vi "BMcalculate_v2_0.vi"() -> ()   [LabVIEW 2014]
uses:
  <vilib>/Analysis/coordinate.llb/2D Cartesian Coordinate Rotation (Array).vi
  <vilib>/Analysis/baseanly.llb/Mean (DBL).vi
  <vilib>/Utility/file.llb/Read From Spreadsheet File (string).vi
  <vilib>/Utility/file.llb/Write To Spreadsheet File (DBL).vi
  <vilib>/Analysis/NI_AALBase.lvlib
  <vilib>/Analysis/NI_AALPro.lvlib
panel:
  in  "(T=X , F=Y)":bool=TRUE
  in  "Filter window size":i32=100
  out "Array":dbl[](array[numeric])
  out "XYplot":path
  out "TimeTrace":path
  in  "Save Time-trace":bool
  in  "nm/pixel":dbl=72.5 format="%#_13g"
  in  "Folder path":path
  in  "?":bool
  in  "to":dbl=1.15 format="%#_13g"
  in  "x/y for all":dbl=0.85 format="%#_13g"
  out "filename":string
  in  "Filter mode":T1(ring)=enum."Median_slide window"
  in  "Save to vertical data ?":bool
  in  "?":enum32{"slide by slide", "delay"}(tab)=enum."delay"
  in  "?":bool
  in  "seconds to wait":u32
  in  "?":dbl=7.963 format="%#_13g"
  in  "?":dbl=48.61 format="%#_13g"
  in  "Save BM":bool
  in  "?":bool=TRUE
  in  "Save X-Y plot":bool
  in  "less than":dbl=0.2 format="%#_13g"
  in  "?":bool
  in  "?":bool
  in  "?":bool=TRUE
  in  "?":T2(tab)
  out "Filenames":string[](array[string])
  out "useful AOIs":i32[](array[numeric])
  out "# of AOI":i32[](array[numeric])
  out "% of useful AOIs":dbl
  out "tt # of AOIs":i32
  out "# of Frames":dbl[](array[numeric])
  out "tt # 0f useful AOIs":i32
  out "?":T3(graph)
  out "size(s)":i32
  out "X-Y plot":cluster{dbl[], dbl[]}(graph)
  out "Xstd":dbl
  out "ystd":dbl[](array[numeric])
  out "X":dbl format="%0.2f"
  out "Y":dbl format="%0.2f"
  out "?":T3(graph)
  out "tt # of useful AOIs":i32
  out "xstd":dbl[](array[numeric])
  out "# of AOI":i32
  out "y 2":dbl[](array[numeric])
  out "# of frames":dbl
  out "all y position (pixel)":dbl[][](array[numeric])
  out "all x position (pixel)":dbl[][](array[numeric])
  out "y":dbl[](array[numeric])
  out "x":dbl[](array[numeric])
  out "y":dbl[](array[numeric])
  out "x":dbl[](array[numeric])
  out "number":dbl[][](array[numeric])
  out "all rows":string[][](array[string])
  out "Useful aoi number":string[][](array[string])
  in  "Tab Control":enum32{"Time trace"}(tab)
  out "Time trace":T4(graph)
  in  "Highlight":dbl=30.0
  in  "±":dbl=30.0
  out "aoi":string
  in  "stop frame1":dbl
  in  "start frame1":dbl
  in  "start frame3":dbl
  in  "stop frame2":dbl
  in  "stop frame3":dbl
  in  "start frame2":dbl
  # "Critiria"
  # "±"
  # "nm"
  # "for ssDNA strande exchange \n                    23.776±6.613 nm"
  # "for D-loop  (90+4)\n                    48.61±7.963 nm"
  # "for D-loop  (150+4)\n                    49.57±8.56 nm"
  # "nm"
  # "Buffer wash"
  # "to"
  # "to"
  # "to"
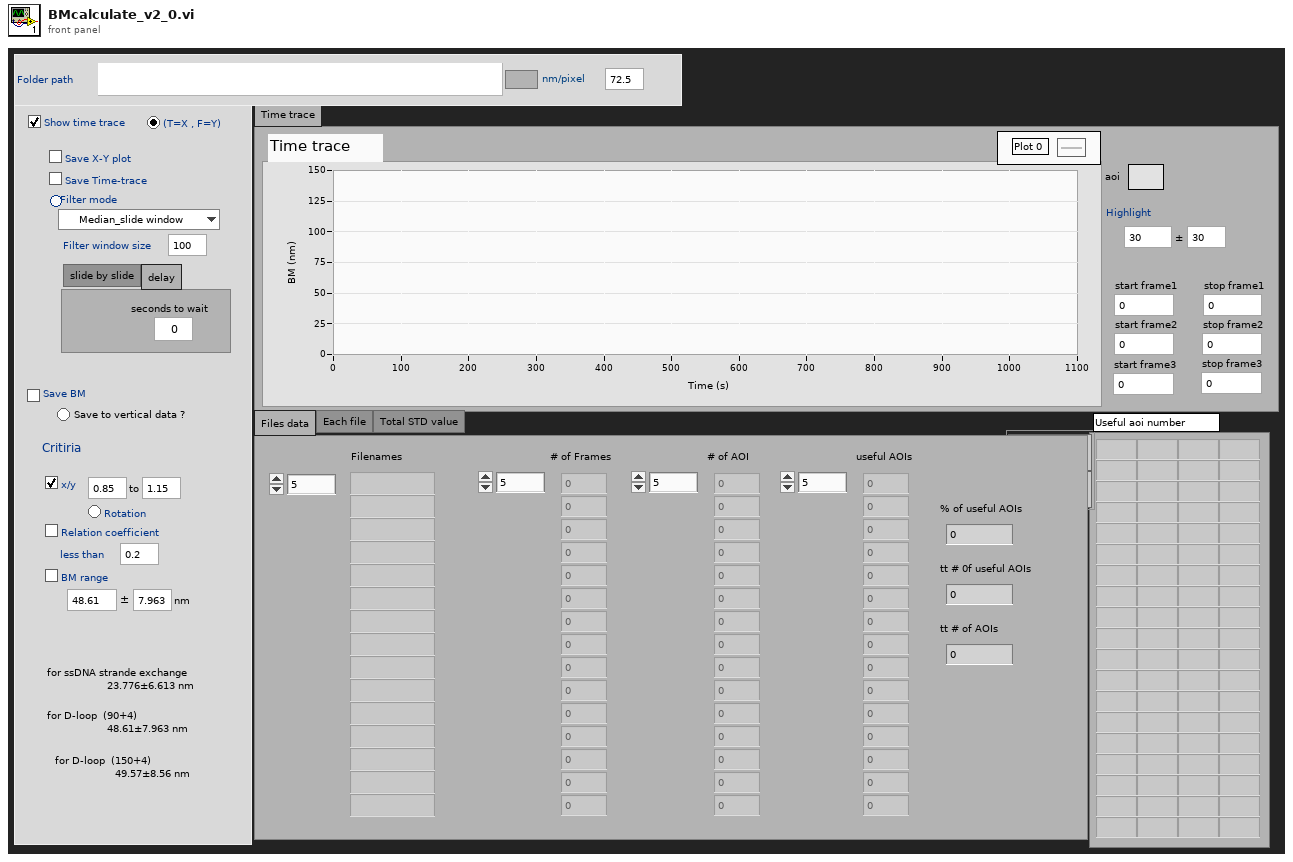
[diagram p1: front panel]
types:
  T1 = enum16{"Median_fix window", "Average_fix window", "Median_slide window", "Average_slide window"}
  T2 = enum32{"Files data", "Each file", "Total STD value"}
  T3 = cluster{"X Values":dbl[], "Histogram: h(x)":i32[]}
  T4 = cluster{"Filtered X":dbl[], "Filtered X":dbl[]}[]
  T5 = cluster{"all y position (pixel)":dbl[], "all x position (pixel)":dbl[]}
  T6 = cluster{"all x position (pixel)":dbl[], "all y position (pixel)":dbl[]}
  T7 = typedef "imagedata.ctl" = cluster{"image type":i32, "image depth":i32, "image":u8[], "mask":u8[], "colors":u32[], "Rectangle":cluster{"left":i16, "top":i16, "right":i16, "bottom":i16}}
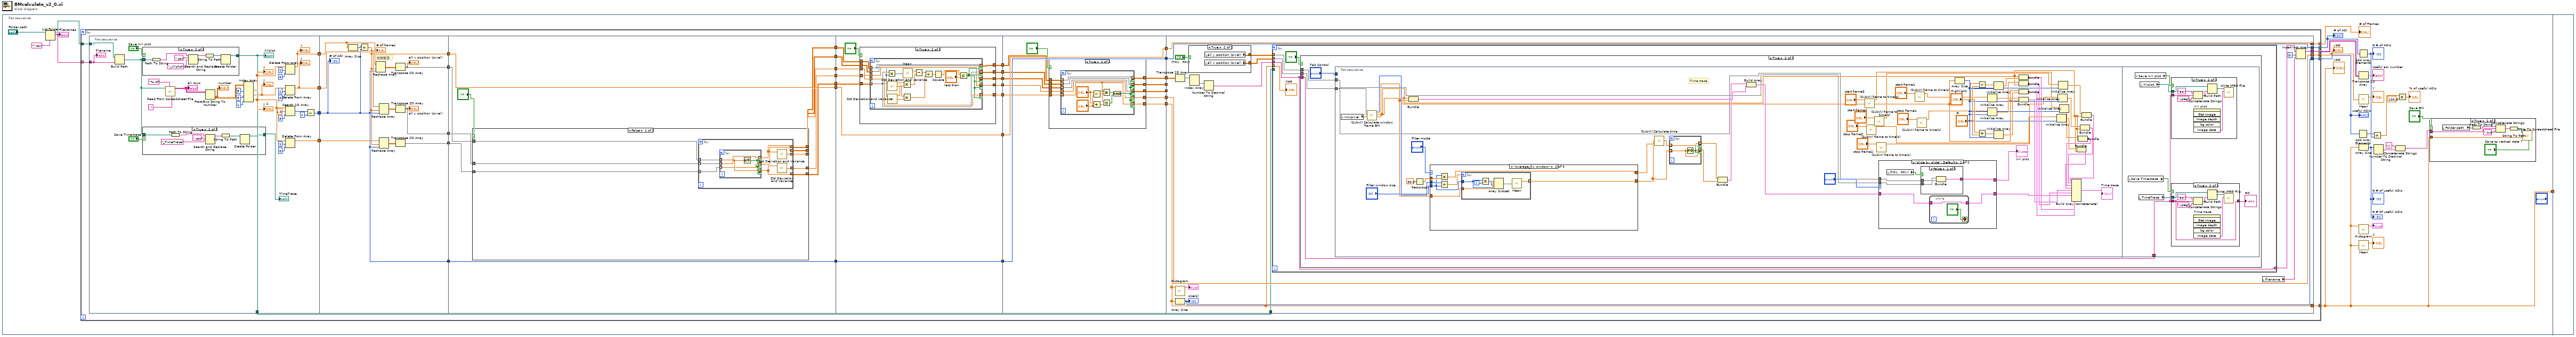
[diagram p0: block diagram]
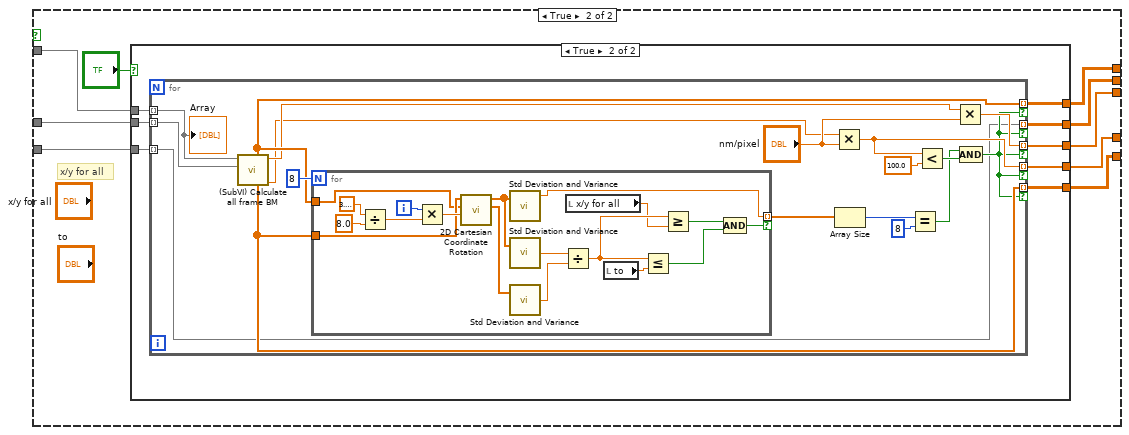
[diagram p5: hidden frame]
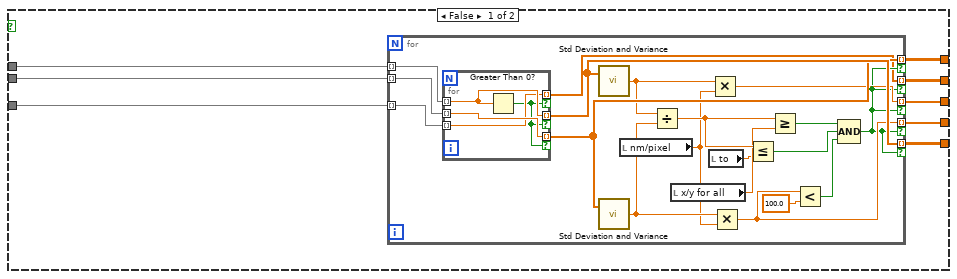
[diagram p6: hidden frame]
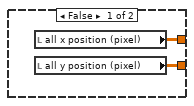
[diagram p9: hidden frame]
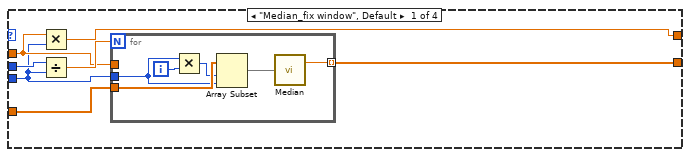
[diagram p11: hidden frame]
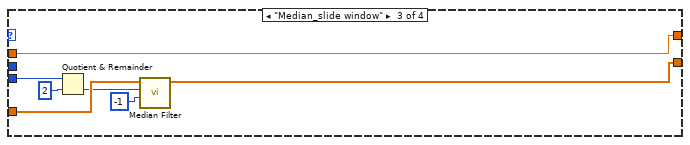
[diagram p12: hidden frame]
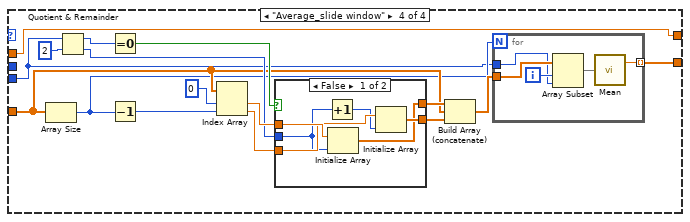
[diagram p13: hidden frame]
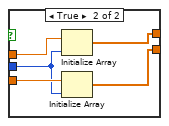
[diagram p14: hidden frame]
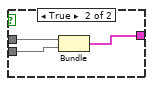
[diagram p15: hidden frame]
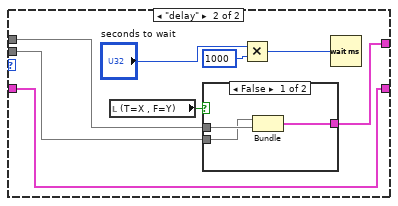
[diagram p16: hidden frame]
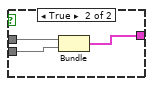
[diagram p17: hidden frame]
diagram:
  n1 = flat-sequence {
    tunnel: [w2] -> w1
    tunnel: w1 -> [_]
    frame #0 {
      n2 = List Folder(path="Folder path", pattern="*.csv") -> (path out=w24:path, filenames=w23:string[])  [unwired: 2 in, 2 out]
      "Filenames" <- w23
      n3 = for {
        tunnel: w24 -> [w37]
        tunnel: w23 -> [w72] mode=indexing
        tunnel: [w71] -> w2 mode=concatenating
        tunnel: [w70] -> w21 mode=indexing
        tunnel: [w69] -> w20 mode=indexing
        tunnel: [w68] -> w12 mode=concatenating
        tunnel: [w67] -> w13 mode=indexing
        tunnel: [w34] -> w4 mode=indexing
        n4 = flat-sequence {
          tunnel: [w92] -> w66
          tunnel: [w91] -> w65
          tunnel: [w85] -> w64
          tunnel: w37 -> [w80]
          tunnel: w72 -> [w76]
          tunnel: [w81] -> w41
          tunnel: [w79] -> w35
          tunnel: w66 -> [w128]
          tunnel: w65 -> [w127]
          tunnel: w64 -> [w126]
          tunnel: [w125] -> w63
          tunnel: [w126] -> w62
          tunnel: [w121] -> w61
          tunnel: [w120] -> w60
          tunnel: w41 -> [w124]
          tunnel: [w122] -> w40
          tunnel: w63 -> [w142]
          tunnel: w62 -> [w141]
          tunnel: w61 -> [w140]
          tunnel: w60 -> [w139]
          tunnel: [w141] -> w53
          tunnel: [w142] -> w51
          tunnel: [w137] -> w49
          tunnel: [w136] -> w47
          tunnel: [w135] -> w45
          tunnel: [w134] -> w43
          tunnel: w40 -> [w132]
          tunnel: [w133] -> w39
          tunnel: w53 -> [w259]
          tunnel: [w259] -> w52
          tunnel: w51 -> [w258]
          tunnel: [w258] -> w50
          tunnel: w49 -> [w254]
          tunnel: [w249] -> w48
          tunnel: w47 -> [w257]
          tunnel: [w252] -> w46
          tunnel: w45 -> [w256]
          tunnel: [w251] -> w44
          tunnel: w43 -> [w255]
          tunnel: [w250] -> w42
          tunnel: w39 -> [w248]
          tunnel: [w247] -> w38
          tunnel: w52 -> [w305]
          tunnel: w50 -> [w304]
          tunnel: w48 -> [w299]
          tunnel: [w305] -> w59
          tunnel: [w304] -> w58
          tunnel: [w298] -> w57
          tunnel: [w302] -> w56
          tunnel: w46 -> [w303]
          tunnel: [w300] -> w55
          tunnel: w44 -> [w301]
          tunnel: [w293] -> w54
          tunnel: w42 -> [w294]
          tunnel: w38 -> [w296]
          tunnel: [w295] -> w36
          tunnel: [w350] -> w68
          tunnel: [w351] -> w67
          tunnel: [w352] -> w69
          tunnel: [w348] -> w70
          tunnel: [w342] -> w71
          tunnel: w59 -> [w352]
          tunnel: w58 -> [w351]
          tunnel: w57 -> [w350]
          tunnel: w56 -> [_]
          tunnel: w55 -> [_]
          tunnel: w54 -> [w342]
          tunnel: w36 -> [w347]
          tunnel: w35 -> [w343]
          tunnel: [w338] -> w34
          frame #0 {
            n5 = Build Path(base path=w80, name or relative path=w76) -> (appended path=w74:path)
            n6 = case shown="True" "Save X-Y plot" {
              tunnel: w74 -> [w112 w119]
              tunnel: [w112 w113] -> w79
              frame False {
              }
              frame True {
                n7 = Path To String(path=w119) -> (string=w118:string)
                n8 = Search and Replace String(input string=w118, search string=".csv", replace string="_XYplot" ("replace string (\"\")")) -> (result string=w115:string)  [unwired: 5 in, 3 out]
                n9 = String To Path(string=w115) -> (path=w114:path)
                n10 = Create Folder(path (use dialog)=w114) -> (created path=w113:path)  [unwired: 2 in, 2 out]
              }
            }
            "XYplot" <- w79
            n11 = case shown="True" "Save Time-trace" {
              tunnel: w74 -> [w104 w111]
              tunnel: [w104 w105] -> w73
              frame False {
              }
              frame True {
                n12 = Path To String(path=w111) -> (string=w110:string)
                n13 = Search and Replace String(input string=w110, search string=".csv", replace string="_TimeTrace" ("replace string (\"\")")) -> (result string=w107:string)  [unwired: 5 in, 3 out]
                n14 = String To Path(string=w107) -> (path=w106:path)
                n15 = Create Folder(path (use dialog)=w106) -> (created path=w105:path)  [unwired: 2 in, 2 out]
              }
            }
            "TimeTrace" <- w73
            n16 = call-poly <vilib>:"Read From Spreadsheet File.vi"("delimiter (\\t)"="," ("delimiter (\\t)"), "format (%s)"="%.4f" ("format (%.3f)"), "file path (dialog if empty)"=w74) -> ("all rows"=w102:string[][])  [unwired: 4 in, 4 out]
            "all rows" <- w102
            n17 = Fract/Exp String To Number(string=w102) -> (number=w101:dbl[][])  [unwired: 3 in, 1 out]
            "number" <- w101
            n18 = Index Array(array=w101, index (col) #1=8 ("disabled index (col)"), index (col) #2=9 ("index (col)"), index (col) #3=1 ("index (col)")) -> (element #1=w93:dbl[], element #2=w94:dbl[], element #3=w82:dbl[])  [unwired: 3 in]
            "x" <- w93
            "y" <- w94
            "y 2" <- w82
            n19 = Delete From Array(array=w93, length=1, index=0) -> (array with subset deleted=w92:dbl[])  [unwired: 1 out]
            "x" <- w92
            n20 = Delete From Array(array=w94, length=1, index=0) -> (array with subset deleted=w91:dbl[])  [unwired: 1 out]
            "y" <- w91
            n21 = Search 1D Array(1D array=w82, element=1.0, start index (0)=3) -> (index of element=w87:i32)
            n22 = Delete From Array(array=w82, length=1, index=0) -> (array with subset deleted=w81:dbl[])  [unwired: 1 out]
            n23 = Subtract(x=w87, y=1) -> (x-y=w85:i32)
            "filename" <- w76
          }
          frame #1 {
            # "矩陣整理"
            n24 = Array Size(array=w128) -> (size(s)=w129:i32)
            n25 = Divide(x=w129, y=w126) -> (x/y=w125:dbl)
            "# of frames" <- w125
            n26 = Reshape Array(w128, w125, w126) -> (w130:dbl[][])
            n27 = Reshape Array(w127, w125, w126) -> (w131:dbl[][])
            n28 = Reshape Array(w124, w125, w126) -> (w123:dbl[][])
            n29 = Transpose 2D Array(2D array=w130) -> (transposed array=w121:dbl[][])
            "all x position (pixel)" <- w121
            n30 = Transpose 2D Array(2D array=w131) -> (transposed array=w120:dbl[][])
            "all y position (pixel)" <- w120
            n31 = Transpose 2D Array(2D array=w123) -> (transposed array=w122:dbl[][])
            "# of AOI" <- w126
          }
          frame #2 {
            n32 = case shown="False" "?" {
              tunnel: [w148 w171] -> w136
              tunnel: [w147 w170] -> w135
              tunnel: w140 -> [w150 w169]
              tunnel: w139 -> [w149 w168]
              tunnel: [w146 w167] -> w134
              tunnel: [w145 w166] -> w137
              tunnel: w132 -> [w144 w164]
              tunnel: [w143 w163] -> w133
              frame False {
                n33 = for {
                  tunnel: w150 -> [w158] mode=indexing
                  tunnel: w149 -> [w157] mode=indexing
                  tunnel: [w156] -> w148 mode=indexing
                  tunnel: [w155] -> w147 mode=indexing
                  tunnel: [w154] -> w146 mode=indexing
                  tunnel: [w153] -> w145 mode=indexing
                  tunnel: w144 -> [w152] mode=indexing
                  tunnel: [w151] -> w143 mode=indexing
                  n34 = for {
                    tunnel: w158 -> [w161] mode=indexing
                    tunnel: w157 -> [w162] mode=indexing
                    tunnel: [w161] -> w156 mode=indexing if=w159
                    tunnel: [w162] -> w155 mode=indexing if=w159
                    tunnel: w152 -> [w160] mode=indexing
                    tunnel: [w160] -> w151 mode=indexing if=w159
                    n35 = Greater Or Equal To 0?(x=w161) -> (x >= 0?=w159:bool)
                  }
                  n36 = call <vilib>:"Std Deviation and Variance.vi"("X"=w155) -> ("standard deviation"=w153:dbl)  [unwired: 1 in, 2 out]
                  n37 = call <vilib>:"Std Deviation and Variance.vi"("X"=w156) -> ("standard deviation"=w154:dbl)  [unwired: 1 in, 2 out]
                }
              }
              frame True {
                # "x/y for all"
                n38 = case shown="True" "?" {
                  tunnel: w168 -> [w178 w210]
                  tunnel: w169 -> [w179 w209]
                  tunnel: [w177 w208] -> w171
                  tunnel: [w176 w207] -> w170
                  tunnel: [w175 w206] -> w167
                  tunnel: [w174 w205] -> w166
                  tunnel: w164 -> [w173 w204]
                  tunnel: [w172 w203] -> w163
                  frame False {
                    n39 = for {
                      tunnel: w179 -> [w198] mode=indexing
                      tunnel: w178 -> [w197] mode=indexing
                      tunnel: [w196] -> w177 mode=indexing if=w183
                      tunnel: [w195] -> w176 mode=indexing if=w183
                      tunnel: [w184] -> w175 mode=indexing if=w183
                      tunnel: [w187] -> w174 mode=indexing if=w183
                      tunnel: [w181] -> w172 mode=indexing if=w183
                      tunnel: w173 -> [w182] mode=indexing
                      n40 = for {
                        tunnel: w198 -> [w201] mode=indexing
                        tunnel: w197 -> [w202] mode=indexing
                        tunnel: [w201] -> w196 mode=indexing if=w199
                        tunnel: [w202] -> w195 mode=indexing if=w199
                        tunnel: w182 -> [w200] mode=indexing
                        tunnel: [w200] -> w181 mode=indexing if=w199
                        n41 = Greater Than 0?(x=w201) -> (x > 0?=w199:bool)
                      }
                      n42 = call <vilib>:"Std Deviation and Variance.vi"("X"=w196) -> ("standard deviation"=w188:dbl)  [unwired: 1 in, 2 out]
                      n43 = call <vilib>:"Std Deviation and Variance.vi"("X"=w195) -> ("standard deviation"=w189:dbl)  [unwired: 1 in, 2 out]
                      n44 = local read "nm/pixel"() -> (w180:dbl)
                      n45 = Divide(x=w188, y=w189) -> (x/y=w194:dbl)
                      n46 = local read "x/y for all"() -> (w193:dbl)
                      n47 = local read "to"() -> (w192:dbl)
                      n48 = Multiply(x=w188, y=w180) -> (x*y=w187:dbl)
                      n49 = Multiply(x=w189, y=w180) -> (x*y=w184:dbl)
                      n50 = Less Or Equal?(x=w194, y=w192) -> (x <= y?=w190:bool)
                      n51 = Greater Or Equal?(x=w194, y=w193) -> (x >= y?=w191:bool)
                      n52 = Less?(x=w184, y=100.0) -> (x < y?=w185:bool)
                      n53 = Compound Arithmetic op=AND(w191, w190, w185) -> (w183:bool)
                    }
                  }
                  frame True {
                    n54 = for {
                      tunnel: w209 -> [w228] mode=indexing
                      tunnel: w210 -> [w227] mode=indexing
                      tunnel: [w214] -> w206 mode=indexing if=w213
                      tunnel: [w221] -> w207 mode=indexing if=w213
                      tunnel: [w222] -> w208 mode=indexing if=w213
                      tunnel: [w219] -> w205 mode=indexing if=w213
                      tunnel: [w211] -> w203 mode=indexing if=w213
                      tunnel: w204 -> [w211] mode=indexing
                      n55 = call "(SubVI) Calculate all frame BM.vi"("y position (pixel)"=w227, "x position (pixel)"=w228) -> ("y standard deviation"=w212:dbl, "x standard deviation"=w220:dbl, "y position (delete y fit error)"=w222:dbl[], "x position (delete x fit error)"=w221:dbl[])  [unwired: 6 in]
                      n56 = for {
                        N: 8 -> [_]
                        tunnel: w222 -> [w241]
                        tunnel: w221 -> [w240]
                        tunnel: [w232] -> w223 mode=indexing if=w231
                        i -> [w242]
                        n57 = Divide(x=3.141592653589793, y=8.0) -> (x/y=w245:dbl)
                        n58 = Multiply(x=w242, y=w245) -> (x*y=w243:dbl)
                        n59 = call-poly <vilib>:"2D Cartesian Coordinate Rotation.vi"("theta"=w243, "Y"=w240, "X"=w241) -> ("Y Out"=w233:dbl[], "X Out"=w234:dbl[])  [unwired: 6 in, 1 out]
                        n60 = call <vilib>:"Std Deviation and Variance.vi"("X"=w234) -> ("mean"=w232:dbl)  [unwired: 1 in, 2 out]
                        n61 = call <vilib>:"Std Deviation and Variance.vi"("X"=w234) -> ("standard deviation"=w239:dbl)  [unwired: 1 in, 2 out]
                        n62 = call <vilib>:"Std Deviation and Variance.vi"("X"=w233) -> ("standard deviation"=w238:dbl)  [unwired: 1 in, 2 out]
                        n63 = Divide(x=w239, y=w238) -> (x/y=w237:dbl)
                        n64 = local read "x/y for all"() -> (w230:dbl)
                        n65 = local read "to"() -> (w229:dbl)
                        n66 = Less Or Equal?(x=w237, y=w229) -> (x <= y?=w235:bool)
                        n67 = Greater Or Equal?(x=w237, y=w230) -> (x >= y?=w236:bool)
                        n68 = Compound Arithmetic op=AND(w236, w235) -> (w231:bool)
                      }
                      n69 = Multiply(x=w212, y="nm/pixel") -> (x*y=w214:dbl)
                      n70 = Array Size(array=w223) -> (size(s)=w225:i32)
                      n71 = Equal?(x=w225, y=8) -> (x = y?=w215:bool)
                      n72 = Less?(x=w214, y=100.0) -> (x < y?=w216:bool)
                      n73 = Multiply(x=w220, y="nm/pixel") -> (x*y=w219:dbl)
                      n74 = Compound Arithmetic op=AND(w215, w216) -> (w213:bool)
                      "Array" <- w228
                    }
                  }
                }
              }
            }
          }
          frame #3 {
            n75 = case shown="True" "?" {
              tunnel: w257 -> [w264 w274]
              tunnel: w256 -> [w263 w273]
              tunnel: w255 -> [w262 w270]
              tunnel: w254 -> [w261 w268]
              tunnel: [w264 w272] -> w252
              tunnel: [w263 w271] -> w251
              tunnel: [w262 w269] -> w250
              tunnel: [w261 w267] -> w249
              tunnel: w248 -> [w260 w266]
              tunnel: [w260 w265] -> w247
              frame False {
              }
              frame True {
                n76 = for {
                  tunnel: w274 -> [w280] mode=indexing
                  tunnel: w273 -> [w279] mode=indexing
                  tunnel: [w280] -> w272 mode=indexing if=w275
                  tunnel: [w279] -> w271 mode=indexing if=w275
                  tunnel: [w287] -> w269 mode=indexing if=w275
                  tunnel: w270 -> [w287] mode=indexing
                  tunnel: w268 -> [w286] mode=indexing
                  tunnel: [w286] -> w267 mode=indexing if=w275
                  tunnel: [w276] -> w265 mode=indexing if=w275
                  tunnel: w266 -> [w276] mode=indexing
                  n77 = Multiply(x=w280, y=w279) -> (x*y=w278:dbl[])
                  n78 = call <vilib>:"Std Deviation and Variance.vi"("X"=w280) -> ("mean"=w283:dbl, "standard deviation"=w285:dbl)  [unwired: 1 in, 1 out]
                  n79 = call <vilib>:"Std Deviation and Variance.vi"("X"=w279) -> ("mean"=w282:dbl, "standard deviation"=w284:dbl)  [unwired: 1 in, 1 out]
                  n80 = Multiply(x=w283, y=w282) -> (x*y=w281:dbl)
                  n81 = Multiply(x=w285, y=w284) -> (x*y=w288:dbl)
                  n82 = call-poly <vilib>:"Mean.vi"("X"=w278) -> ("mean"=w277:dbl)  [unwired: 1 out]
                  n83 = Subtract(x=w277, y=w281) -> (x-y=w289:dbl)
                  n84 = Divide(x=w289, y=w288) -> (x/y=w290:dbl)
                  n85 = Square(x=w290) -> (x^2=w291:dbl)
                  n86 = Less Or Equal?(x=w291, y="less than") -> (x <= y?=w275:bool)
                }
              }
            }
          }
          frame #4 {
            n87 = case shown="True" "?" {
              tunnel: [w311 w321] -> w302
              tunnel: w303 -> [w311 w322]
              tunnel: w301 -> [w310 w320]
              tunnel: [w310 w319] -> w300
              tunnel: w294 -> [w309 w318]
              tunnel: [w309 w317] -> w293
              tunnel: w299 -> [w308 w316]
              tunnel: [w308 w315] -> w298
              tunnel: w296 -> [w307 w314]
              tunnel: [w306 w313] -> w295
              frame False {
                n88 = for {
                  tunnel: w307 -> [w312] mode=indexing
                  tunnel: [w312] -> w306 mode=indexing
                }
              }
              frame True {
                n89 = for {
                  tunnel: [w334] -> w321 mode=indexing if=w329
                  tunnel: w322 -> [w334] mode=indexing
                  tunnel: [w333] -> w319 mode=indexing if=w329
                  tunnel: w320 -> [w333] mode=indexing
                  tunnel: [w323] -> w317 mode=indexing if=w329
                  tunnel: w318 -> [w323] mode=indexing
                  tunnel: w316 -> [w328] mode=indexing
                  tunnel: [w328] -> w315 mode=indexing if=w329
                  tunnel: [w330] -> w313 mode=indexing if=w329
                  tunnel: w314 -> [w330] mode=indexing
                  n90 = Subtract(x="?", y="?") -> (x-y=w325:dbl)
                  n91 = Add(x="?", y="?") -> (x+y=w324:dbl)
                  n92 = Greater Or Equal?(x=w323, y=w325) -> (x >= y?=w332:bool)
                  n93 = Less Or Equal?(x=w323, y=w324) -> (x <= y?=w331:bool)
                  n94 = Compound Arithmetic op=AND(w332, w331) -> (w329:bool)
                }
              }
            }
          }
          frame #5 {
            n95 = Transpose 2D Array(2D array=w347) -> (transposed array=w346:dbl[][])
            n96 = call <vilib>:"Histogram.vi"("X"=w342) -> ("Histogram Graph"=→"?":T3)  [unwired: 7 in, 3 out]
            n97 = Array Size(array=w342) -> (size(s)=w348:i32)
            "size(s)" <- w348
            n98 = case shown="True" "(T=X , F=Y)" {
              tunnel: [w354 w356] -> w336
              tunnel: [w353 w355] -> w335
              frame False {
                n99 = local read "all x position (pixel)"() -> (w353:dbl[][])
                n100 = local read "all y position (pixel)"() -> (w354:dbl[][])
              }
              frame True {
                n101 = local read "all y position (pixel)"() -> (w355:dbl[][])
                n102 = local read "all x position (pixel)"() -> (w356:dbl[][])
              }
            }
            n103 = Index Array(array=w346) -> (element=w345:dbl[])  [unwired: 2 in]
            n104 = Number To Decimal String(number=w345) -> (decimal integer string=w344:string[])  [unwired: 1 in]
            n105 = for {
              tunnel: w336 -> [w360] mode=indexing
              tunnel: w335 -> [w361] mode=indexing
              tunnel: w344 -> [w357] mode=indexing
              tunnel: w343 -> [_]
              tunnel: w342 -> [w358] mode=indexing
              tunnel: [w357] -> w339 mode=indexing
              n106 = case shown="True" "?" {
                tunnel: w361 -> [_ w365]
                tunnel: w360 -> [_ w364]
                tunnel: w357 -> [_ w363]
                frame False {
                }
                frame True {
                  n107 = flat-sequence {
                    tunnel: w365 -> [w411]
                    tunnel: w364 -> [w410]
                    tunnel: "Tab Control" -> [_]
                    tunnel: w363 -> [w521]
                    frame #0 {
                      # "Time trace"
                      n108 = local read "nm/pixel"() -> (w400:dbl)
                      n109 = call "(SubVI) Calculate window frame BM.vi"("nm/pixel"=w400, "all x position (pixel)"=w410) -> ("BM"=w395:dbl[], "sec"=w382:dbl[], "frame"=w416:i32)  [unwired: 3 in]
                      n110 = Bundle("sec"=w382, "BM"=w395) -> (w415:cluster{"sec":dbl[], "BM":dbl[]})  [unwired: 1 in]
                      n111 = Reciprocal(x=30.0) -> (1/x=w397:dbl)
                      n112 = case shown="\"Average_fix window\"" "Filter mode" {
                        tunnel: [w429 w440 w455 w472] -> w394
                        tunnel: w395 -> [w430 w441 w456 w461]
                        tunnel: w416 -> [w428 w443 _ _]
                        tunnel: "Filter window size" -> [w424 w437 w452 w458]
                        tunnel: w397 -> [w426 w439 w454 w457]
                        tunnel: [w425 w438 w454 w457] -> w396
                        frame "Median_fix window", Default {
                          n113 = Multiply(x=w426, y=w424) -> (x*y=w425:dbl)
                          n114 = Divide(x=w428, y=w424) -> (x/y=w427:dbl)
                          n115 = for {
                            N: w427 -> [_]
                            tunnel: w430 -> [w436]
                            tunnel: [w434] -> w429 mode=indexing
                            tunnel: w424 -> [w431]
                            tunnel: w426 -> [_]
                            i -> [w433]
                            n116 = Multiply(x=w431, y=w433) -> (x*y=w432:i32)
                            n117 = Array Subset(array=w436, index=w432, length=w431) -> (w435:dbl[])
                            n118 = call <vilib>:"Median.vi"("X"=w435) -> ("median"=w434:dbl)  [unwired: 1 out]
                          }
                        }
                        frame "Average_fix window" {
                          n119 = Multiply(x=w437, y=w439) -> (x*y=w438:dbl)
                          n120 = Divide(x=w443, y=w437) -> (x/y=w442:dbl)
                          n121 = for {
                            N: w442 -> [_]
                            tunnel: w441 -> [w449]
                            tunnel: [w447] -> w440 mode=indexing
                            tunnel: w437 -> [w445]
                            i -> [w446]
                            n122 = Multiply(x=w445, y=w446) -> (x*y=w444:i32)
                            n123 = Array Subset(array=w449, index=w444, length=w445) -> (w448:dbl[])
                            n124 = call-poly <vilib>:"Mean.vi"("X"=w448) -> ("mean"=w447:dbl)  [unwired: 1 out]
                          }
                        }
                        frame "Median_slide window" {
                          n125 = Quotient & Remainder(x=w452, y=2) -> (floor(x/y)=w450:i32)  [unwired: 1 out]
                          n126 = call <vilib>:"Median Filter.vi"("right rank"=-1, "left rank"=w450, "X"=w456) -> ("Filtered X"=w455:dbl[])  [unwired: 7 in, 1 out]
                        }
                        frame "Average_slide window" {
                          n127 = Array Size(array=w461) -> (size(s)=w459:i32)
                          n128 = Quotient & Remainder(x=w458, y=2) -> (x-y*floor(x/y)=w468:i32, floor(x/y)=w466:i32)
                          n129 = Equal To 0?(x=w468) -> (x = 0?=w467:bool)
                          n130 = Decrement(x=w459) -> (x-1=w465:i32)
                          n131 = Index Array(array=w461, index #1=0 ("index"), index #2=w465) -> (element #1=w470:dbl, element #2=w464:dbl)
                          n132 = case shown="False" w467 {
                            tunnel: w470 -> [w478 w483]
                            tunnel: w466 -> [w475 w481]
                            tunnel: w464 -> [w477 w482]
                            tunnel: [w473 w480] -> w463
                            tunnel: [w474 w479] -> w462
                            frame False {
                              n133 = Increment(x=w475) -> (x+1=w476:i32)
                              n134 = Initialize Array(w478, w475) -> (w473:dbl[])
                              n135 = Initialize Array(w477, w476) -> (w474:dbl[])
                            }
                            frame True {
                              n136 = Initialize Array(w483, w481) -> (w480:dbl[])
                              n137 = Initialize Array(w482, w481) -> (w479:dbl[])
                            }
                          }
                          n138 = Build Array (concatenate)(w463, w461, w462) -> (w460:dbl[])
                          n139 = for {
                            N: w459 -> [_]
                            tunnel: w460 -> [w488]
                            tunnel: [w486] -> w472 mode=indexing
                            tunnel: w458 -> [w484]
                            i -> [w485]
                            n140 = Array Subset(array=w488, index=w485, length=w484) -> (w487:dbl[])
                            n141 = call-poly <vilib>:"Mean.vi"("X"=w487) -> ("mean"=w486:dbl)  [unwired: 1 out]
                          }
                        }
                      }
                      n142 = call "(SubVI) Calculate time.vi"("dt"=w396, "BM"=w394) -> ("Time (s)"=w393:dbl[])  [unwired: 3 in]
                      n143 = for {
                        tunnel: w394 -> [w421] mode=indexing
                        tunnel: [w421] -> w391 mode=indexing if=w422
                        tunnel: w393 -> [w423] mode=indexing
                        tunnel: [w423] -> w392 mode=indexing if=w422
                        n144 = Not Equal To 0?(x=w421) -> (x != 0?=w422:bool)
                      }
                      n145 = Bundle(w392, w391) -> (w420:cluster{dbl[], dbl[]})  [unwired: 1 in]
                      n146 = Build Array(w420, w415) -> (w419:cluster{"sec":dbl[], "BM":dbl[]}[])
                      n147 = call "(SubVI) frame to time(s).vi"("Numeric in"="start frame3") -> ("Numeric out"=w367:dbl)  [unwired: 10 in]
                      n148 = call "(SubVI) frame to time(s).vi"("Numeric in"="stop frame3") -> ("Numeric out"=w366:dbl)  [unwired: 10 in]
                      n149 = call "(SubVI) frame to time(s).vi"("Numeric in"="start frame2") -> ("Numeric out"=w371:dbl)  [unwired: 10 in]
                      n150 = call "(SubVI) frame to time(s).vi"("Numeric in"="stop frame2") -> ("Numeric out"=w370:dbl)  [unwired: 10 in]
                      n151 = case shown="\"slide by slide\", Default" "?" {
                        tunnel: w419 -> [w494 w510]
                        tunnel: [w493 w510] -> w412
                        tunnel: w410 -> [w492 w506]
                        tunnel: w411 -> [w491 w505]
                        tunnel: [w490 w504] -> w414
                        frame "slide by slide", Default {
                          n152 = local read "(T=X , F=Y)"() -> (w489:bool)
                          n153 = case shown="False" w489 {
                            tunnel: w492 -> [w497 w500]
                            tunnel: w491 -> [w496 w499]
                            tunnel: [w495 w498] -> w490
                            frame False {
                              n154 = Bundle("all y position (pixel)"=w496, "all x position (pixel)"=w497) -> (w495:T5)  [unwired: 1 in]
                            }
                            frame True {
                              n155 = Bundle("all x position (pixel)"=w500, "all y position (pixel)"=w499) -> (w498:T6)  [unwired: 1 in]
                            }
                          }
                          n156 = while {
                            tunnel: w494 -> [w501]
                            tunnel: [w501] -> w493
                            stop <- "?" stop-if-true
                          }
                        }
                        frame "delay" {
                          n157 = local read "(T=X , F=Y)"() -> (w503:bool)
                          n158 = case shown="False" w503 {
                            tunnel: w506 -> [w513 w516]
                            tunnel: w505 -> [w512 w515]
                            tunnel: [w511 w514] -> w504
                            frame False {
                              n159 = Bundle("all y position (pixel)"=w512, "all x position (pixel)"=w513) -> (w511:T5)  [unwired: 1 in]
                            }
                            frame True {
                              n160 = Bundle("all x position (pixel)"=w516, "all y position (pixel)"=w515) -> (w514:T6)  [unwired: 1 in]
                            }
                          }
                          n161 = Multiply(x="seconds to wait", y=u32 1000) -> (x*y=w508:u32)
                          n162 = Wait (ms)(milliseconds to wait=w508) -> ()  [unwired: 1 out]
                        }
                      }
                      "X-Y plot" <- w414
                      n163 = call "(SubVI) frame to time(s).vi"("Numeric in"="start frame1") -> ("Numeric out"=w377:dbl)  [unwired: 10 in]
                      n164 = call "(SubVI) frame to time(s).vi"("Numeric in"="stop frame1") -> ("Numeric out"=w374:dbl)  [unwired: 10 in]
                      n165 = Array Size(array=w382) -> (size(s)=w388:i32)
                      n166 = Subtract(x="Highlight", y="±") -> (x-y=w404:dbl)
                      n167 = Add(x="Highlight", y="±") -> (x+y=w403:dbl)
                      n168 = Initialize Array(w377, w388) -> (w402:dbl[])
                      n169 = Initialize Array(w374, w388) -> (w401:dbl[])
                      n170 = Initialize Array(w404, w388) -> (w409:dbl[])
                      n171 = Initialize Array(w403, w388) -> (w408:dbl[])
                      n172 = Bundle("sec"=w382, w409) -> (w413:cluster{"sec":dbl[], dbl[]})  [unwired: 1 in]
                      n173 = Bundle(w401, "sec"=w382) -> (w389:cluster{dbl[], "sec":dbl[]})  [unwired: 1 in]
                      n174 = Bundle("sec"=w382, w408) -> (w407:cluster{"sec":dbl[], dbl[]})  [unwired: 1 in]
                      n175 = Bundle(w402, "sec"=w382) -> (w390:cluster{dbl[], "sec":dbl[]})  [unwired: 1 in]
                      n176 = Initialize Array(w366, w388) -> (w383:dbl[])
                      n177 = Initialize Array(w370, w388) -> (w385:dbl[])
                      n178 = Initialize Array(w371, w388) -> (w386:dbl[])
                      n179 = Initialize Array(w367, w388) -> (w384:dbl[])
                      n180 = Bundle(w383, "sec"=w382) -> (w378:cluster{dbl[], "sec":dbl[]})  [unwired: 1 in]
                      n181 = Bundle(w384, "sec"=w382) -> (w379:cluster{dbl[], "sec":dbl[]})  [unwired: 1 in]
                      n182 = Bundle(w385, "sec"=w382) -> (w380:cluster{dbl[], "sec":dbl[]})  [unwired: 1 in]
                      n183 = Bundle(w386, "sec"=w382) -> (w381:cluster{dbl[], "sec":dbl[]})  [unwired: 1 in]
                      n184 = Build Array (concatenate)(w381, w380, w379, w378, w390, w389, w412, w413, w407) -> (→"Time trace":cluster{"sec":dbl[], "BM":dbl[]}[])
                    }
                    frame #1 {
                      n185 = local read "Save Time-trace"() -> (w522:bool)
                      n186 = local read "Save X-Y plot"() -> (w519:bool)
                      n187 = local read "TimeTrace"() -> (w520:path)
                      n188 = local read "XYplot"() -> (w518:path)
                      n189 = case shown="True" w519 {
                        tunnel: w521 -> [_ w529]
                        tunnel: w518 -> [_ w526]
                        frame False {
                        }
                        frame True {
                          n190 = Concatenate Strings("aoi" ("string"), w529, ".jpeg" ("string")) -> (w527:string)
                          n191 = invoke on="X-Y plot" class="XYGraph (strict)" method="Get Image"() -> ("image data"=w524:T7)  [unwired: 6 in, 5 out]
                          n192 = Build Path(base path=w526, name or relative path=w527) -> (appended path=w525:path)
                          n193 = call <vilib>:"Write JPEG File.vi"("image data"=w524, "path to JPEG file"=w525) -> ()  [unwired: 8 in, 2 out]
                        }
                      }
                      n194 = case shown="True" w522 {
                        tunnel: w521 -> [w530 w532]
                        tunnel: w520 -> [_ w535]
                        tunnel: [w530 w532] -> w517
                        frame False {
                        }
                        frame True {
                          n195 = Concatenate Strings("aoi" ("string"), w532, ".jpeg" ("string")) -> (w536:string)
                          n196 = invoke on="Time trace" class="XYGraph (strict)" method="Get Image"() -> ("image data"=w531:T7)  [unwired: 6 in, 5 out]
                          n197 = Build Path(base path=w535, name or relative path=w536) -> (appended path=w534:path)
                          n198 = call <vilib>:"Write JPEG File.vi"("image data"=w531, "path to JPEG file"=w534) -> ()  [unwired: 8 in, 2 out]
                        }
                      }
                      "aoi" <- w517
                    }
                  }
                }
              }
              "Xstd" <- w358
            }
            n199 = local read "filename"() -> (w341:string)
            n200 = Insert Into Array(array=w339, index=0, new element=w341) -> (w338:string[])
          }
        }
      }
      "useful AOIs" <- w21
      "# of AOI" <- w20
      "ystd" <- w12
      "# of Frames" <- w13
      "xstd" <- w2
      n201 = Add Array Elements(numeric array=w21) -> (sum=w19:i32)
      n202 = Add Array Elements(numeric array=w20) -> (sum=w18:i32)
      "tt # of AOIs" <- w18
      n203 = Transpose 2D Array(2D array=w4) -> (transposed array=→"Useful aoi number":string[][])
      n204 = call-poly <vilib>:"Mean.vi"("X"=w12) -> ("mean"=→"Y":dbl)  [unwired: 1 out]
      n205 = Array Size(array=w2) -> (size(s)=w9:i32)
      "tt # 0f useful AOIs" <- w9
      "tt # of useful AOIs" <- w9
      n206 = call <vilib>:"Histogram.vi"("X"=w2) -> ("Histogram Graph"=→"?":T3)  [unwired: 7 in, 3 out]
      n207 = call-poly <vilib>:"Mean.vi"("X"=w2) -> ("mean"=→"X":dbl)  [unwired: 1 out]
      n208 = Divide(x=w19, y=w18) -> (x/y=w17:dbl)
      n209 = Number To Decimal String(number=w9) -> (decimal integer string=w7:string)  [unwired: 1 in]
      n210 = Concatenate Strings("\\" ("string"), w7) -> (w6:string)
      n211 = Multiply(x=w17, y=100.0) -> (x*y=→"% of useful AOIs":dbl)
      n212 = case shown="True" "Save BM" {
        tunnel: w2 -> [_ w33]
        tunnel: w6 -> [_ w27]
        frame False {
        }
        frame True {
          n213 = local read "Folder path"() -> (w32:path)
          n214 = Path To String(path=w32) -> (string=w31:string)
          n215 = Concatenate Strings(w31, w27, ".txt" ("string")) -> (w30:string)
          n216 = String To Path(string=w30) -> (path=w29:path)
          n217 = call-poly <vilib>:"Write To Spreadsheet File.vi"("transpose? (no:F)"="Save to vertical data ?", "1D data"=w33, "file path (dialog if empty)"=w29) -> ()  [unwired: 5 in, 1 out]
        }
      }
    }
    frame #1 {
    }
  }
